vi "Supported Smart Syntax Representation.vi"(0 "Comparison Operations in":refnum<class "Comparison Functions.lvclass">, 11 "error in (no error)":errorcluster) -> (4 "Comparison Operations out":refnum<class "Comparison Functions.lvclass">, 6 "Smart Syntax Representation List":string[](array[string]), 15 "error out":errorcluster)   [LabVIEW 2019, in "Comparison Functions.lvclass"]
uses:
  Comparison Functions.lvclass
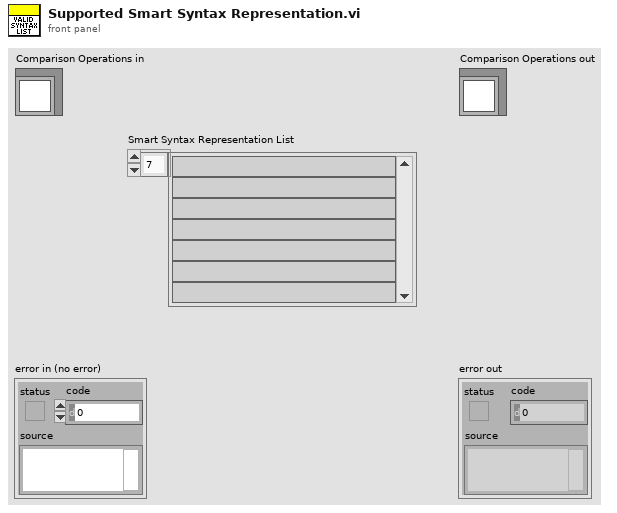
[diagram p1: front panel]
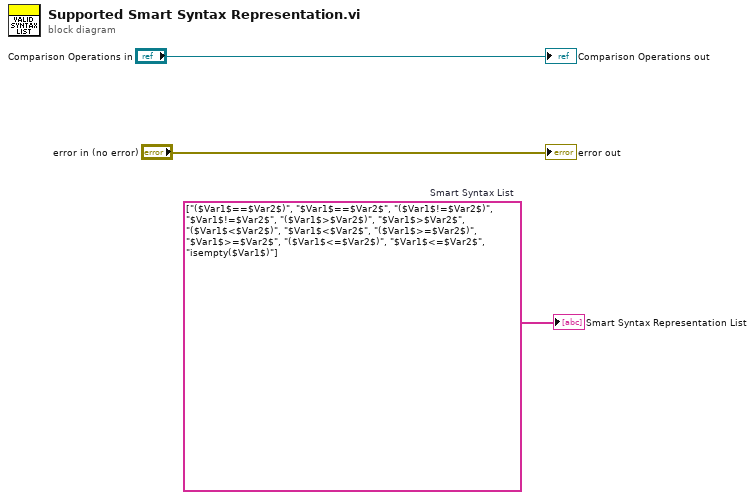
[diagram p0: block diagram]
diagram:
  w1 = string[] ["($Var1$==$Var2$)", "$Var1$==$Var2$", "($Var1$!=$Var2$)", "$Var1$!=$Var2$", "($Var1$>$Var2$)", "$Var1$>$Var2$", "($Var1$<$Var2$)", "$Var1$<$Var2$", "($Var1$>=$Var2$)", "$Var1$>=$Var2$", "($Var1$<=$Var2$)", "$Var1$<=$Var2$", "isempty($Var1$)"]  # Smart Syntax List
  "error out" <- "error in (no error)"
  "Comparison Operations out" <- "Comparison Operations in"
  "Smart Syntax Representation List" <- w1
